vi "fgv_img_u8array.vi"(7 "cmd":enum16{"init", "read", "write"}(ring), 11 "data":u8[](array[numeric])) -> (3 "image array":u8[](array[numeric]))   [LabVIEW 2019]
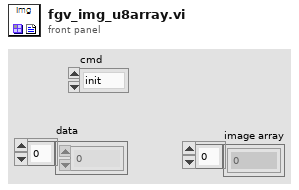
[diagram p1: front panel]
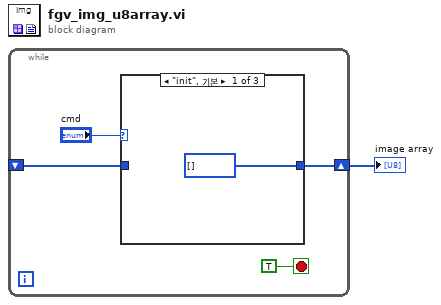
[diagram p0: block diagram]
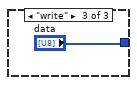
[diagram p3: hidden frame]
diagram:
  n1 = while {
    shift-right: [w3] -> w1
    shift-left: _ -> [w2]
    stop <- TRUE stop-if-true
    n2 = case shown="\"init\", 기본" "cmd" {
      tunnel: [u8[] [] ("Global Rectangle") w7 "data"] -> w3
      tunnel: w2 -> [_ w7 _]
      frame "init", Default {
      }
      frame "read" {
      }
      frame "write" {
      }
    }
  }
  "image array" <- w1
